vi "Union Unified Msg Set.vi"(11 "TEMPLATE Actor in":refnum<class "TEMPLATE Actor.lvclass">) -> (2 "Unified Msg Set":T1)   [LabVIEW 2020, in "_Template.lvlib" / "Templates.lvlib" / "TEMPLATE Actor.lvlib" / "TEMPLATE Actor.lvclass"]
uses:
  TEMPLATE Actor.lvclass
  jettl/jettl/Actor/Msg Set.ctl
  jettl/jettl/Msg/Msg.lvclass
  TEMPLATE Actor.lvclass/TEMPLATE Actor.ctl
  jettl/jettl/Actor/Actor/Actor.lvclass
  jettl/jettl/Actor/Actor.lvlib
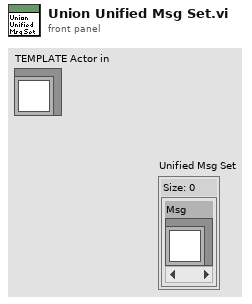
[diagram p1: front panel]
types:
  T1 = typedef "jettl.lvlib/Actor.lvlib/Msg Set.ctl" = set{refnum<class "Msg.lvclass">}
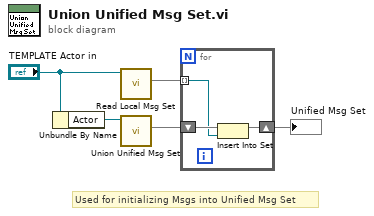
[diagram p0: block diagram]
diagram:
  # "Used for initializing Msgs into Unified Msg Set"
  n1 = Unbundle By Name("TEMPLATE Actor in") -> ("Actor"=w4:refnum<class "Actor.lvclass">)
  n2 = call-dynamic "Read Local Msg Set.vi"("TEMPLATE Actor in"="TEMPLATE Actor in") -> ("Local Msg Set"=w1:T1)  [unwired: 10 in]
  n3 = call-dynamic "Union Unified Msg Set.vi"("Get Actor in"=w4) -> ("Unified Msg Set"=w3:T1)  [unwired: 10 in]
  n4 = for {
    shift-right: [w7] -> w5
    shift-left: w3 -> [w8]
    tunnel: w1 -> [w6] mode=indexing
    n5 = Insert Into Set(10:w6, 11:w8) -> (3:w7:T1)  [unwired: 1 out]
  }
  "Unified Msg Set" <- w5
